vi "Random Image.vi"() -> (2 "Picture":u16(ring), 3 "Random Number":dbl)   [LabVIEW 2014]
doc: "This VI generates a random image from a picture ring."
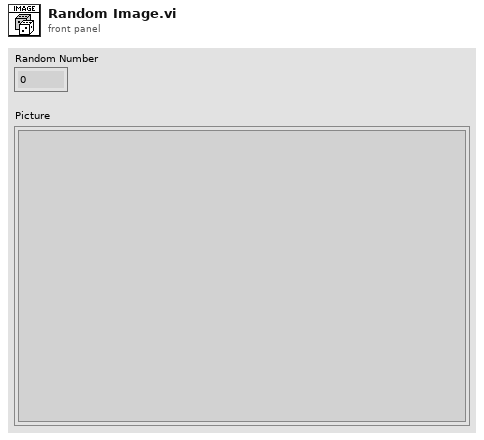
[diagram p1: front panel]
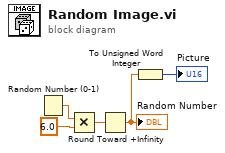
[diagram p0: block diagram]
diagram:
  n1 = Random Number (0-1)() -> (number: 0 to 1=w4:dbl)
  n2 = Multiply(x=w4, y=6.0) -> (x*y=w3:dbl)
  n3 = Round Toward +Infinity(x=w3) -> (ceil(x): smallest int >= x=w1:dbl)
  "Random Number" <- w1
  n4 = To Unsigned Word Integer(number=w1) -> (unsigned 16bit integer=→"Picture":u16)
